vi "ATE_PwrMtr_Cal.vi"() -> ()   [LabVIEW 2009]
doc: "Use this template to build a producer/consumer design pattern with events to produce queue items. Use this design pattern instead of the User Interface Event Handler pattern for user interfaces when you want to execute code asynchronously in response to an event without slowing the user interface responsiveness."
uses:
  <vilib>/Analysis/NI_AALPro.lvlib
panel:
  in  "Sig Gen Test Point":T1(ring)
  out "Mean Diff":dbl format="%0.2f"
  out "Std Dev":dbl format="%0.2f"
  in  "Power Meter Test Point":T2(ring)
  in  "Calibrate-Atten":bool
  in  "Configuration 1":bool
  in  "Set SigGen":bool
  in  "70 dB":bool
  in  "121 dB":bool
  in  "Switches":bool
  in  "Calibrate-SG":bool
  in  "Stop":bool
  out "Output File":path
  out "SigGen - PwrMtr":cluster{dbl[], dbl[]}[](graph)
  out "ATE_Power_Cal":cluster{dbl[], dbl[]}[](graph)
  in  "Data Directory":string="/home/operator/ate/data/ate_cal"
  in  "ATE TABS":enum32{"Status", "Controls"}(tab)=enum."Controls"
  out "ATE Switch Status":T3
  out "121dB\nAttenuators":bool[](array[boolean])
  out "70dB\nAttenuators":bool[](array[boolean])
  out "Signal Generator Status":T4={"Frequency (GHz)"=0.0, "RF Power (dBm)"=0.0, "RF Power"=TRUE} {"RF Power (dBm)" format="%.2g"}
  out "Power (dBm)":dbl
  out "121 Verified":bool
  out "70 Verfied":bool
  out "Power Returned (dBm)":dbl format="%.3f"
  in  "ATE Switches":T5
  in  "121 dB Atten":i32=121 min=0 max=121 step=1
  in  "70 dB Attn":i32=70 min=0 max=70 step=10
  in  "Start dBm":dbl=-5.0
  in  "Steps":i32=21
  in  "Steps Size":dbl=1.0 min=0.1 max=2.0 step=0.1 format="%.1g"
  out "P-State":string
  out "C-State":string
  # "1 dB"
  # "2 dB"
  # "4 dB"
  # "4 dB"
  # "10 dB"
  # "20 dB"
  # "40 dB"
  # "40 dB"
  # "10 dB"
  # "20 dB"
  # "40 dB"
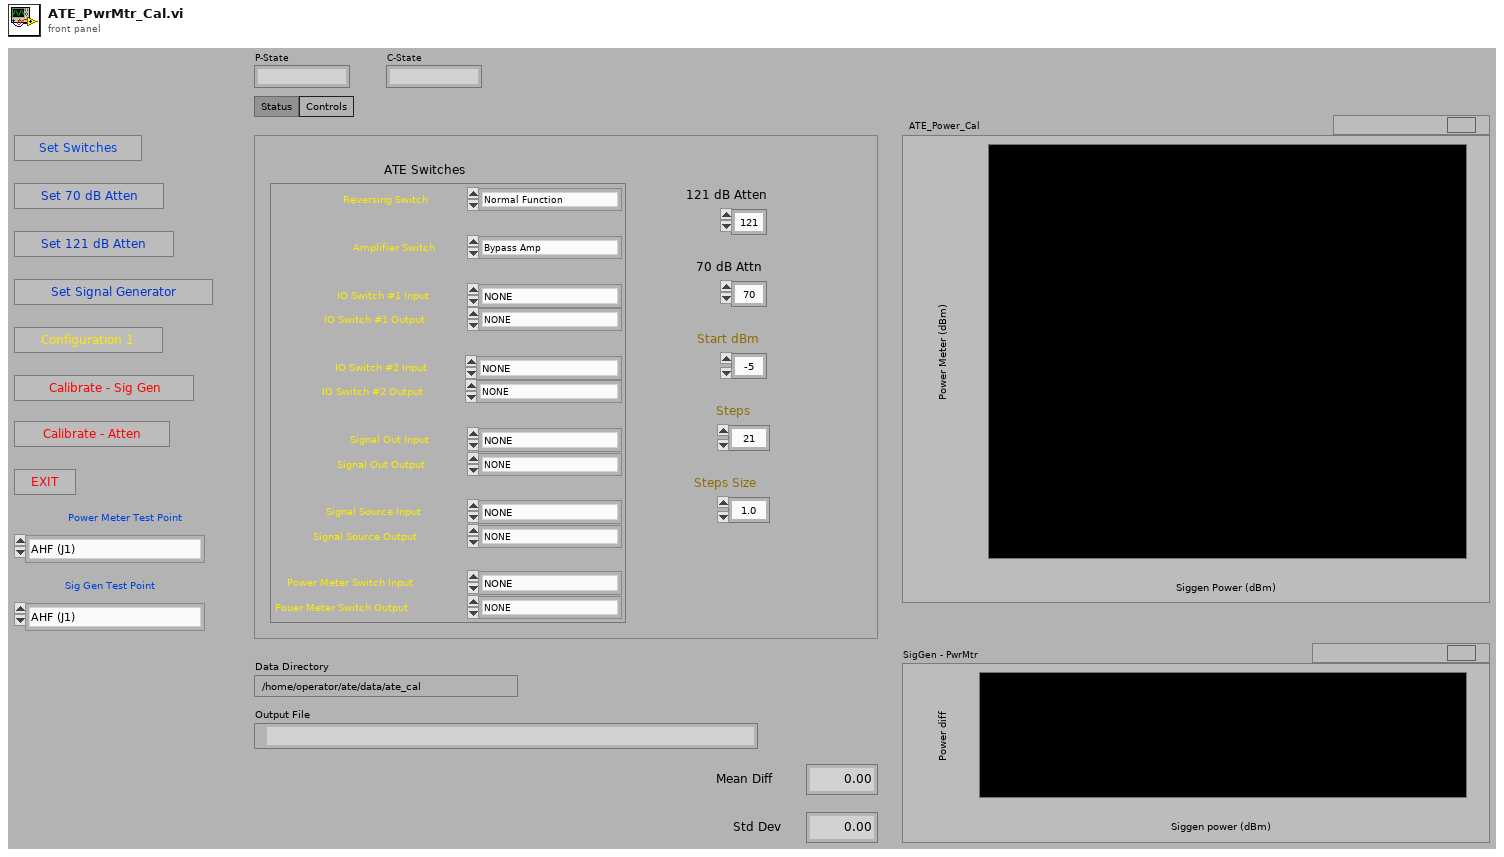
[diagram p1: front panel]
types:
  T1 = enum16{"AHF (J1)", "AHR (J2)", "AVR (J3)", "AVF (J4)", "NG1 (J5)", "Power Meter (J6)", "Sig Gen (J7)", "TXH-TXV Switch (J8)", "Power Meter Direct", ""}
  T2 = enum16{"AHF (J1)", "AHR (J2)", "AVR (J3)", "AVF (J4)", "NG1 (J5)", "Power Meter (J6)", "Sig Gen (J7)", "TXH-TXV Switch (J8)", "Sig Gen Direct"}
  T3 = cluster{"Reversing Switch ":bool, "IO Switch #1":bool, "IO Switch #2":bool, "Signal Out":bool, "Signal Source":bool, "Power Meter":bool, "Amp By Pass":bool}
  T4 = cluster{"Frequency (GHz)":dbl, "RF Power (dBm)":dbl, "RF Power":bool}
  T5 = cluster{"Reversing Switch":enum16{"Normal Function", "Reversing Function"}, "IO Switch #1 Input":enum16{"NONE", "AHR (J2)", "Splitter", "Signal Out Switch (S3)", "Reversing Switch"}, "IO Switch #1 Output":enum16{"NONE", "AHR (J2)", "Delay Device (S4)", "Power Meter Switch (S5)", "Reversing Switch"}, "IO Switch #2 Input":enum16{"NONE", "AVR (J3)", "Splitter", "Signal Out Switch (S3)", " 2W Term (TM1)", "Reversing Switch"}, "IO Switch #2 Output":enum16{"NONE", "AVR (J3)", "Signal Out Switch (S3)", "Power Meter Switch (S5)", "Reversing Switch", "2W Term (TM1)"}, "Signal Out Input":enum16{"NONE", "Amp Bypass Switch (S6)", "IO Switch #1 (S1)", "IO Switch #2 (S2)", "2W Term (TM3)"}, "Signal Out Output":enum16{"NONE", "2 Watt Term (TM3)", "Splitter", "Power Meter Switch (S5)"}, "Signal Source Input":enum16{"NONE", "Delay Device", "Signal Generator (J7)", "Inside Noise Box NF (J5)", "2W Term (TM3)"}, "Signal Source Output":enum16{"NONE", "Amp Bypass Switch", "Test Pulse Generator", "Power Meter Switch (S5)"}, "Power Meter Switch Input":enum16{"NONE", "IO Switch #1 (S1)", "Signal Source Switch (S4)", "Signal Out Switch (S3)", "IO Switch #2 (S2)", "TXH-TXV Switch (J8)"}, "Pouer Meter Switch Output":enum16{"NONE", "Power Meter (J6)"}, "Amplifier Switch":enum16{"Bypass Amp", "Include Amp"}}
  T6 = cluster{"Frequency (GHz)":dbl, "RF Power (dBm)":dbl, "RF ON/OFF":bool}
  T7 = enum16{"open", "replace", "create", "open or create", "replace or create", "replace or create with confirmation"}
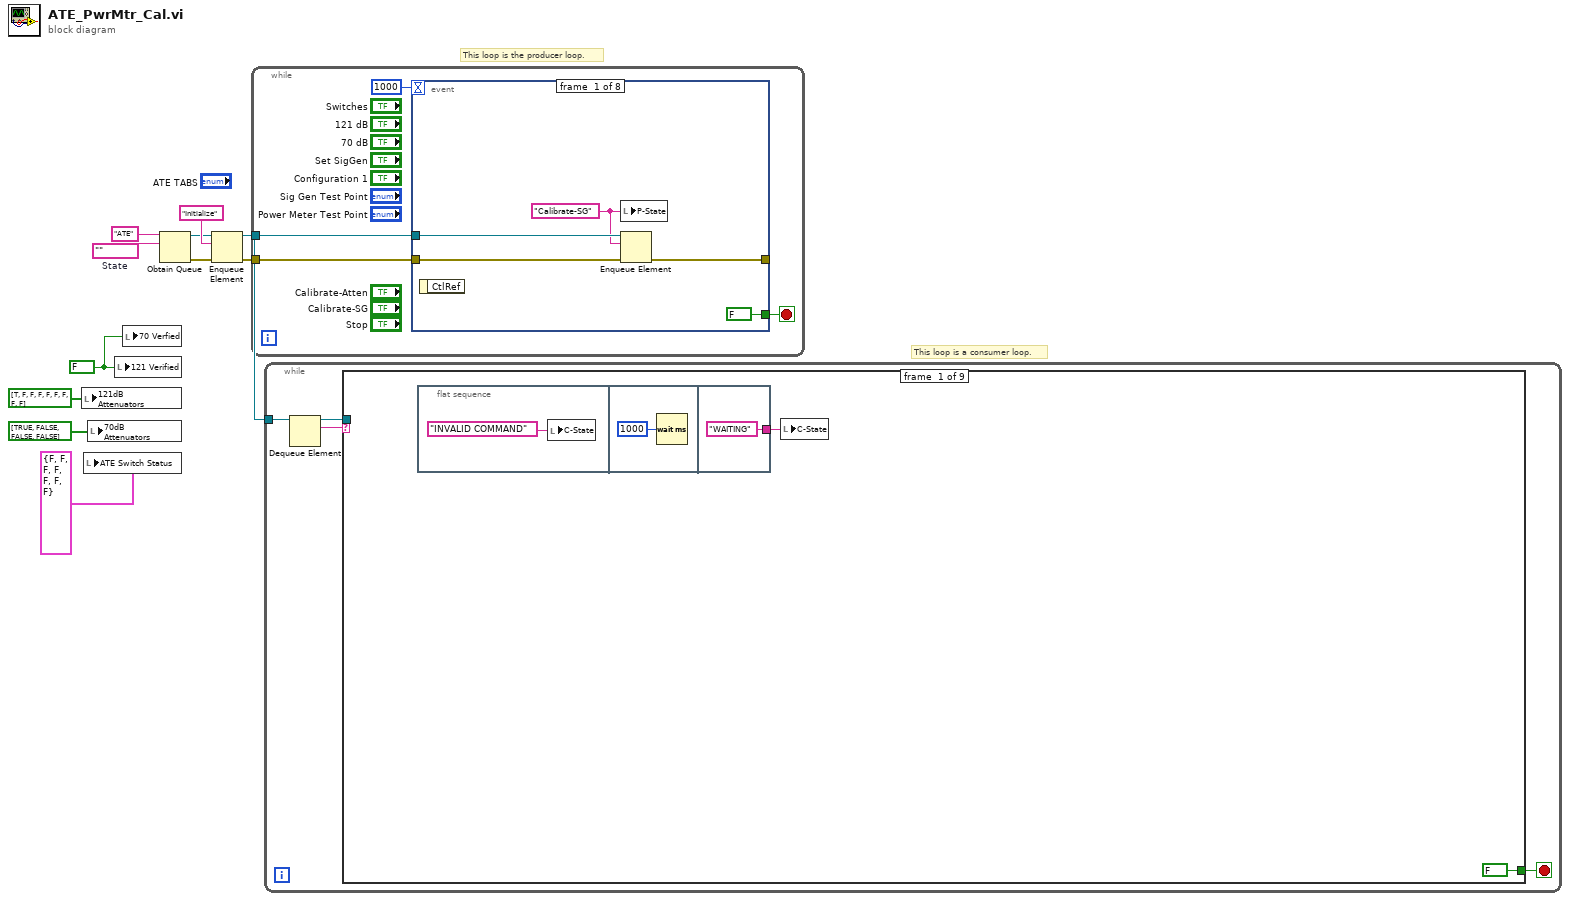
[diagram p0: block diagram]
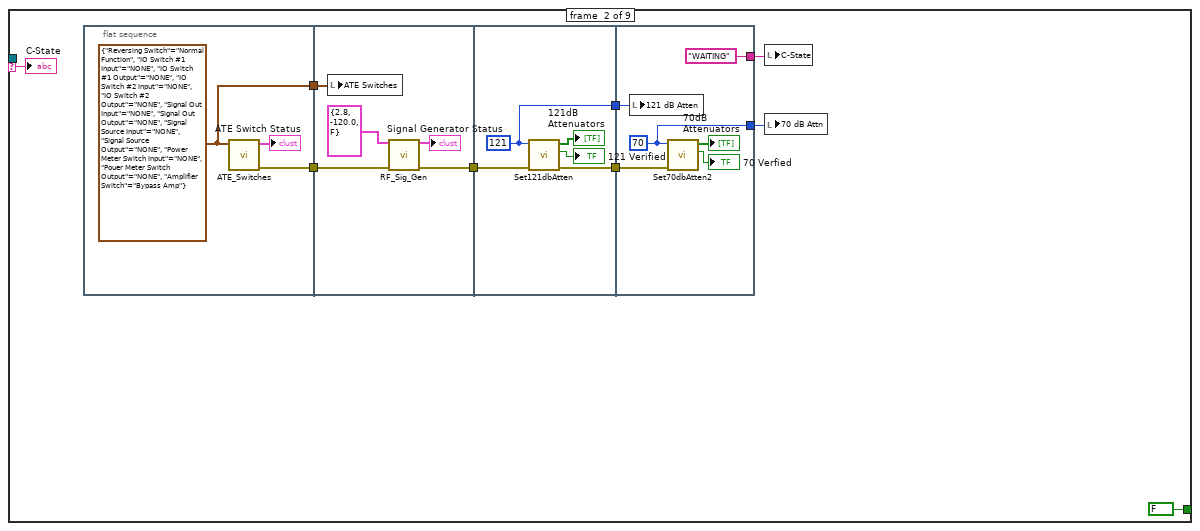
[diagram p2: hidden frame]
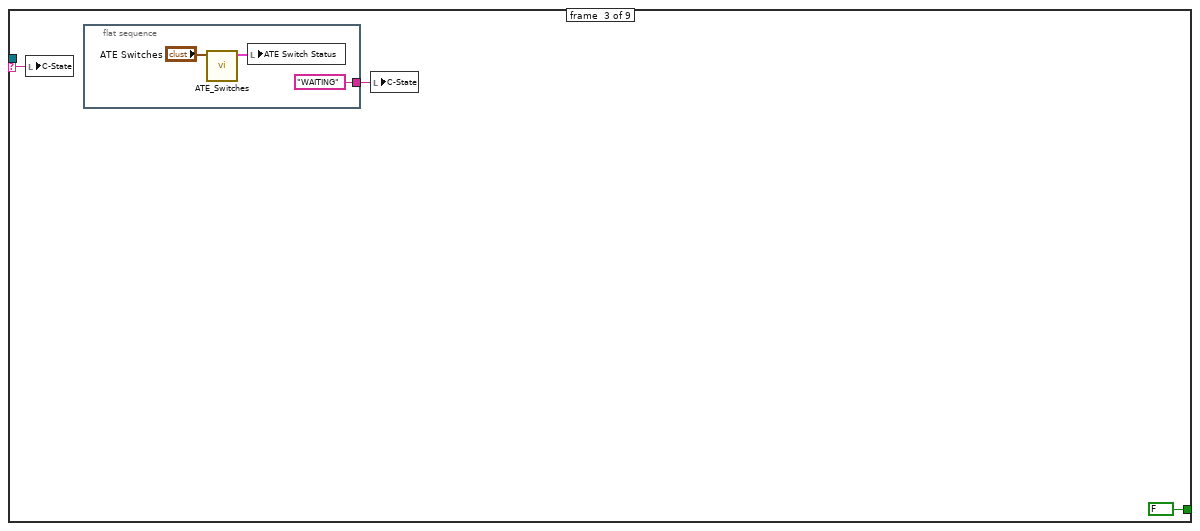
[diagram p3: hidden frame]
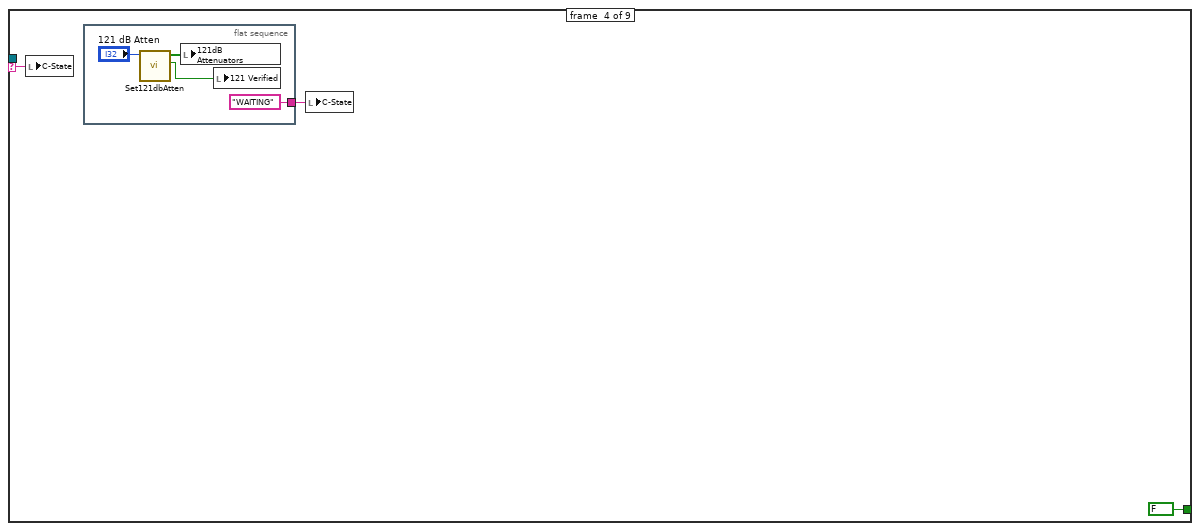
[diagram p4: hidden frame]
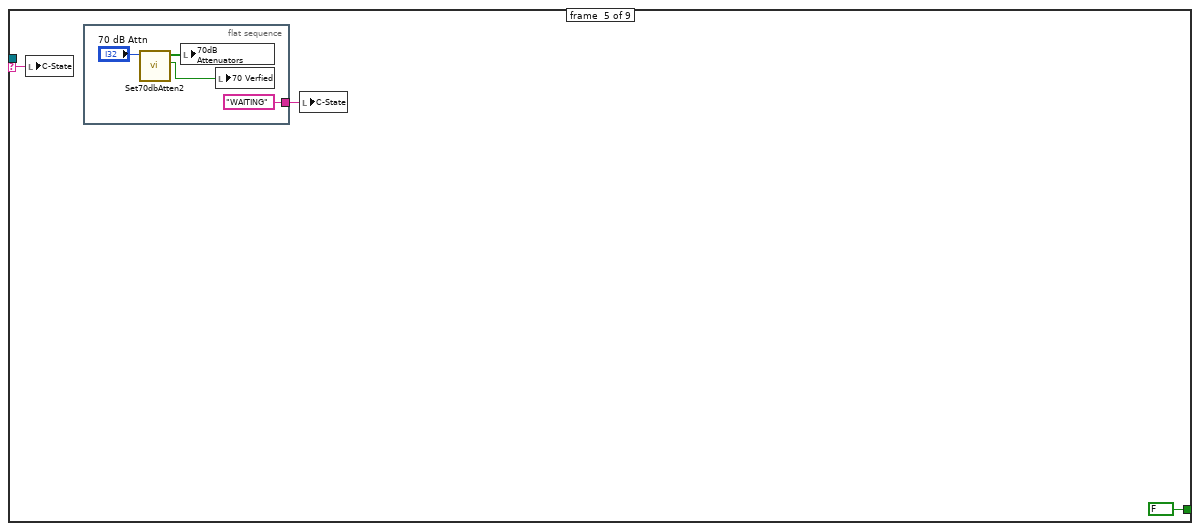
[diagram p5: hidden frame]
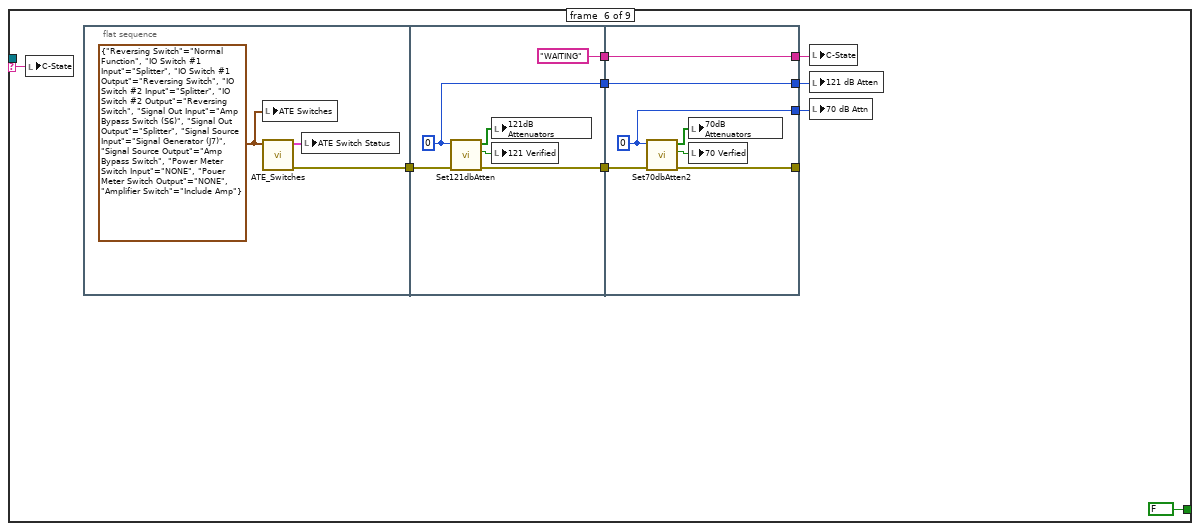
[diagram p6: hidden frame]
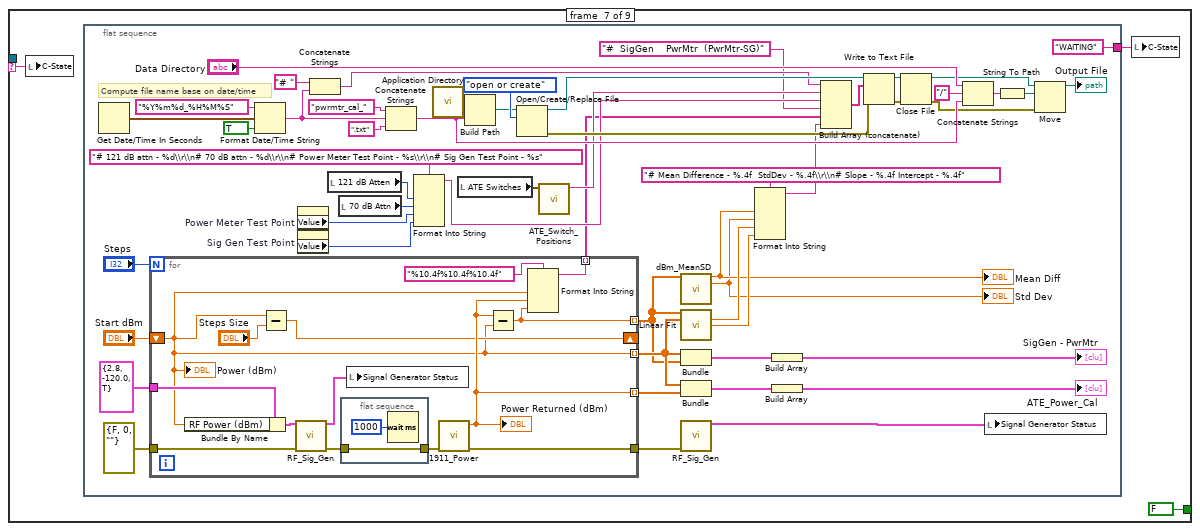
[diagram p7: hidden frame]
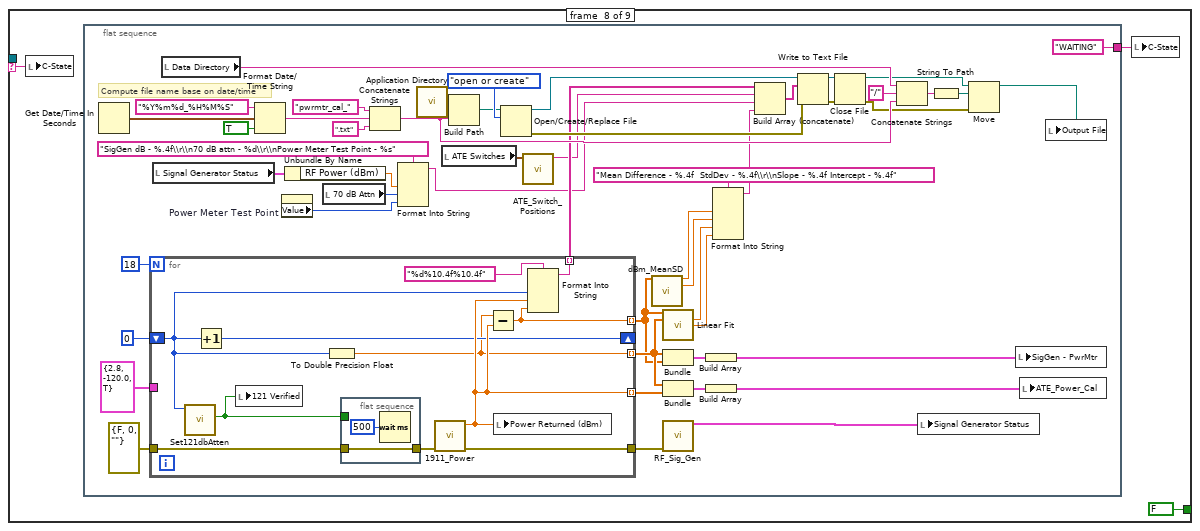
[diagram p8: hidden frame]
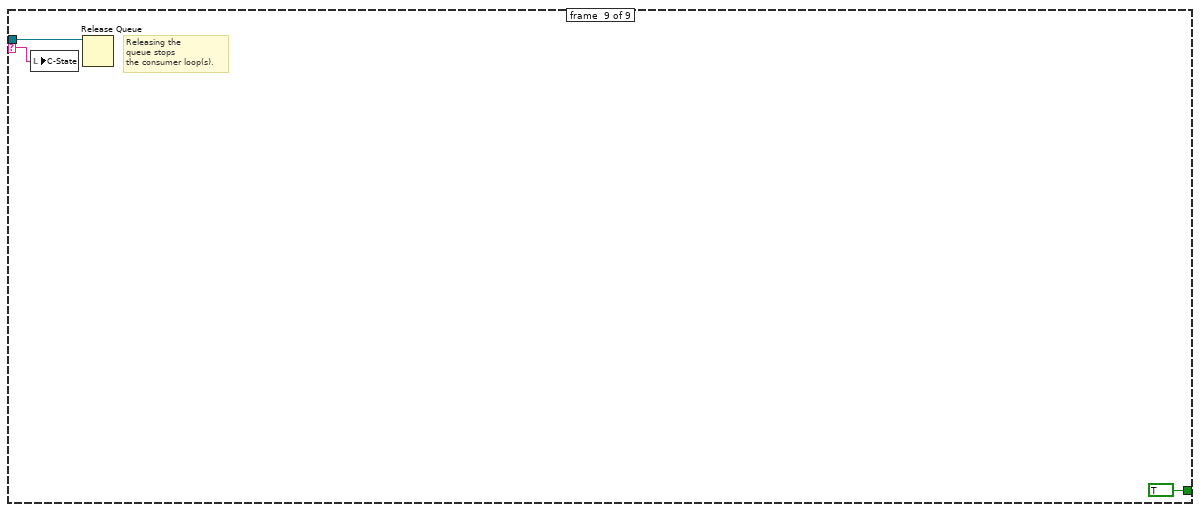
[diagram p9: hidden frame]
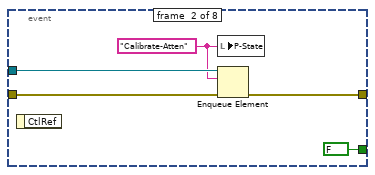
[diagram p10: hidden frame]
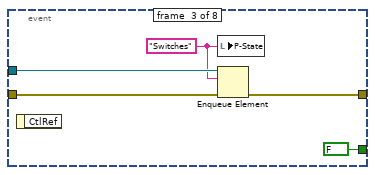
[diagram p11: hidden frame]
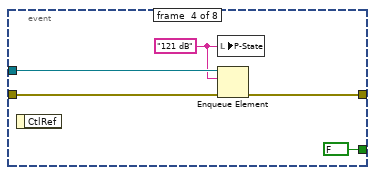
[diagram p12: hidden frame]
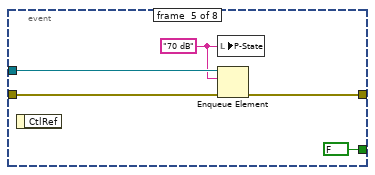
[diagram p13: hidden frame]
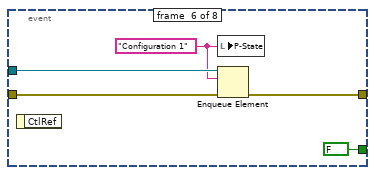
[diagram p14: hidden frame]
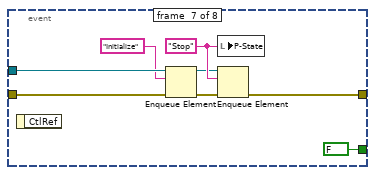
[diagram p15: hidden frame]
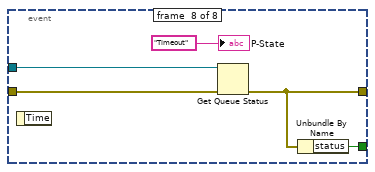
[diagram p16: hidden frame]
diagram:
  w1 = FALSE ("70 Verfied")
  w11 = ""  # State
  # "This loop is the producer loop."
  # "This loop is a consumer loop."
  n1 = local write "121dB\nAttenuators"(bool[] [TRUE, FALSE, FALSE, FALSE, FALSE, FALSE, FALSE, FALSE, FALSE] ("121dB\nAttenuators")) -> ()
  n2 = local write "ATE Switch Status"(T3 {"Reversing Switch "=FALSE, "IO Switch #1"=FALSE, "IO Switch #2"=FALSE, "Signal Out"=FALSE, "Signal Source"=FALSE, "Power Meter"=FALSE, "Amp By Pass"=FALSE} ("ATE Switch Status")) -> ()
  n3 = local write "70dB\nAttenuators"(bool[] [TRUE, FALSE, FALSE, FALSE] ("70dB\nAttenuators")) -> ()
  n4 = local write "121 Verified"(w1) -> ()
  n5 = local write "70 Verfied"(w1) -> ()
  n6 = Obtain Queue(name (unnamed)="ATE", element data type=w11) -> (queue out=w8:refnum<queue>, error out=w6:errorcluster)  [unwired: 3 in, 1 out]
  n7 = Enqueue Element(queue=w8, element="Initialize", error in (no error)=w6) -> (queue out=w7:refnum<queue>, error out=w5:errorcluster)  [unwired: 1 in, 1 out]
  n8 = while {
    tunnel: w7 -> [w15]
    tunnel: w5 -> [w14]
    stop <- w12 stop-if-true
    n9 = event shown="[6] \"Stop\": Value Change" {
      selector: _ -> [_ _ _ _ _ _ _ _]
      dyn-events: _ -> [_ _ _ _ _ _ _ _]
      timeout: 1000 -> [_ _ _ _ _ _ _ _]
      tunnel: w15 -> [w20 w25 w30 w35 w40 w45 w48 w58]
      tunnel: w14 -> [w19 w24 w29 w34 w39 w44 w50 w54]
      tunnel: [w18 w23 w28 w33 w38 w43 w53 w56] -> _
      tunnel: [FALSE FALSE FALSE FALSE FALSE FALSE FALSE w57] -> w12
      event #0 {
        w16 = "Calibrate-SG" ("element")
        n10 = event-data() -> ()  [unwired: 1 in, 1 out]
        n11 = local write "P-State"(w16) -> ()
        n12 = Enqueue Element(queue=w20, element=w16, error in (no error)=w19) -> (error out=w18:errorcluster)  [unwired: 1 in, 2 out]
      }
      event #1 {
        w21 = "Calibrate-Atten" ("element")
        n13 = event-data() -> ()  [unwired: 1 in, 1 out]
        n14 = local write "P-State"(w21) -> ()
        n15 = Enqueue Element(queue=w25, element=w21, error in (no error)=w24) -> (error out=w23:errorcluster)  [unwired: 1 in, 2 out]
      }
      event #2 {
        w26 = "Switches" ("element")
        n16 = event-data() -> ()  [unwired: 1 in, 1 out]
        n17 = local write "P-State"(w26) -> ()
        n18 = Enqueue Element(queue=w30, element=w26, error in (no error)=w29) -> (error out=w28:errorcluster)  [unwired: 1 in, 2 out]
      }
      event #3 {
        w31 = "121 dB" ("element")
        n19 = event-data() -> ()  [unwired: 1 in, 1 out]
        n20 = local write "P-State"(w31) -> ()
        n21 = Enqueue Element(queue=w35, element=w31, error in (no error)=w34) -> (error out=w33:errorcluster)  [unwired: 1 in, 2 out]
      }
      event #4 {
        w36 = "70 dB" ("element")
        n22 = event-data() -> ()  [unwired: 1 in, 1 out]
        n23 = local write "P-State"(w36) -> ()
        n24 = Enqueue Element(queue=w40, element=w36, error in (no error)=w39) -> (error out=w38:errorcluster)  [unwired: 1 in, 2 out]
      }
      event #5 {
        w41 = "Configuration 1" ("element")
        n25 = event-data() -> ()  [unwired: 1 in, 1 out]
        n26 = local write "P-State"(w41) -> ()
        n27 = Enqueue Element(queue=w45, element=w41, error in (no error)=w44) -> (error out=w43:errorcluster)  [unwired: 1 in, 2 out]
      }
      event #6 {
        w51 = "Stop" ("element")
        n28 = event-data() -> ()  [unwired: 1 in, 1 out]
        n29 = Enqueue Element(queue=w48, element="Initialize", error in (no error)=w50) -> (queue out=w47:refnum<queue>, error out=w49:errorcluster)  [unwired: 1 in, 1 out]
        n30 = local write "P-State"(w51) -> ()
        n31 = Enqueue Element(queue=w47, element=w51, error in (no error)=w49) -> (error out=w53:errorcluster)  [unwired: 1 in, 2 out]
      }
      event #7 {
        n32 = event-data() -> ()  [unwired: 1 in, 1 out]
        n33 = Get Queue Status(queue=w58, error in (no error)=w54) -> (error out=w56:errorcluster)  [unwired: 1 in, 7 out]
        n34 = Unbundle By Name(w56) -> ("status"=w57:bool)
        "P-State" <- "Timeout" ("element")
      }
    }
  }
  n35 = while {
    tunnel: w7 -> [w62]
    stop <- w59 stop-if-true
    n36 = Dequeue Element(queue=w62) -> (queue out=w60:refnum<queue>, element=w61:string)  [unwired: 2 in, 2 out]
    n37 = case shown="\"Calibrate-Atten\"" w61 {
      selector: w61 -> [_ w75 w98 w103 w110 w123 w142 w215 w282]
      tunnel: w60 -> [_ _ _ _ _ _ _ _ w281]
      tunnel: [FALSE FALSE FALSE FALSE FALSE FALSE FALSE FALSE TRUE] -> w59
      frame #0 {
        n38 = flat-sequence {
          tunnel: ["WAITING" ("element")] -> w63
          frame #0 {
            n39 = local write "C-State"("INVALID COMMAND" ("C-State")) -> ()
          }
          frame #1 {
            n40 = Wait (ms)(milliseconds to wait=u32 1000) -> ()  [unwired: 1 out]
          }
          frame #2 {
          }
        }
        n41 = local write "C-State"(w63) -> ()
      }
      frame #1 {
        n42 = flat-sequence {
          tunnel: [w78] -> w72
          tunnel: [w77] -> w70
          tunnel: w72 -> [w82]
          tunnel: [w81] -> w71
          tunnel: w70 -> [w80]
          tunnel: w71 -> [w88]
          tunnel: [w87] -> w73
          tunnel: [w86] -> w69
          tunnel: ["WAITING" ("element")] -> w74
          tunnel: w73 -> [w94]
          tunnel: w69 -> [w92]
          tunnel: [w90] -> w68
          frame #0 {
            w77 = T5 {"Reversing Switch"=enum."Normal Function", "IO Switch #1 Input"=enum."NONE", "IO Switch #1 Output"=enum."NONE", "IO Switch #2 Input"=enum."NONE", "IO Switch #2 Output"=enum."NONE", "Signal Out Input"=enum."NONE", "Signal Out Output"=enum."NONE", "Signal Source Input"=enum."NONE", "Signal Source Output"=enum."NONE", "Power Meter Switch Input"=enum."NONE", "Pouer Meter Switch Output"=enum."NONE", "Amplifier Switch"=enum."Bypass Amp"} ("ATE Switches")
            n43 = call "ATE_Switches.vi"("ATE Switches"=w77) -> ("Switch Errors"=w78:errorcluster, "ATE Switch Status"=→"ATE Switch Status":T3)  [unwired: 9 in]
          }
          frame #1 {
            n44 = local write "ATE Switches"(w80) -> ()
            n45 = call "RF_Sig_Gen.vi"("Signal Generator Control"=T6 {"Frequency (GHz)"=2.8, "RF Power (dBm)"=-120.0, "RF ON/OFF"=FALSE}, "error in"=w82) -> ("Signal Generator Status"=→"Signal Generator Status":T4, "Sig Gen Errors"=w81:errorcluster)  [unwired: 12 in]
          }
          frame #2 {
            w86 = 121 ("Attenuation (dB)")
            n46 = call "Set121dbAtten.vi"("error in (no error)"=w88, "Attenuation (dB)"=w86) -> ("error out"=w87:errorcluster, "Verfied"=→"121 Verified":bool, "Active Attenuators"=→"121dB\nAttenuators":bool[])  [unwired: 7 in]
          }
          frame #3 {
            w90 = 70 ("Attenuation (dB)")
            n47 = local write "121 dB Atten"(w92) -> ()
            n48 = call "Set70dbAtten2.vi"("error in (no error)"=w94, "Attenuation (dB)"=w90) -> ("Verfied"=→"70 Verfied":bool, "Active Attenuators"=→"70dB\nAttenuators":bool[])  [unwired: 7 in, 1 out]
          }
        }
        n49 = local write "C-State"(w74) -> ()
        n50 = local write "70 dB Attn"(w68) -> ()
        "C-State" <- w75
      }
      frame #2 {
        n51 = local write "C-State"(w98) -> ()
        n52 = flat-sequence {
          tunnel: ["WAITING" ("element")] -> w96
          frame #0 {
            n53 = call "ATE_Switches.vi"("ATE Switches"="ATE Switches") -> ("ATE Switch Status"=w100:T3)  [unwired: 9 in, 1 out]
            n54 = local write "ATE Switch Status"(w100) -> ()
          }
        }
        n55 = local write "C-State"(w96) -> ()
      }
      frame #3 {
        n56 = local write "C-State"(w103) -> ()
        n57 = flat-sequence {
          tunnel: ["WAITING" ("element")] -> w102
          frame #0 {
            n58 = call "Set121dbAtten.vi"("Attenuation (dB)"="121 dB Atten") -> ("Verfied"=w105:bool, "Active Attenuators"=w107:bool[])  [unwired: 8 in, 1 out]
            n59 = local write "121dB\nAttenuators"(w107) -> ()
            n60 = local write "121 Verified"(w105) -> ()
          }
        }
        n61 = local write "C-State"(w102) -> ()
      }
      frame #4 {
        n62 = local write "C-State"(w110) -> ()
        n63 = flat-sequence {
          tunnel: ["WAITING" ("element")] -> w109
          frame #0 {
            n64 = call "Set70dbAtten2.vi"("Attenuation (dB)"="70 dB Attn") -> ("Verfied"=w112:bool, "Active Attenuators"=w114:bool[])  [unwired: 8 in, 1 out]
            n65 = local write "70dB\nAttenuators"(w114) -> ()
            n66 = local write "70 Verfied"(w112) -> ()
          }
        }
        n67 = local write "C-State"(w109) -> ()
      }
      frame #5 {
        n68 = local write "C-State"(w123) -> ()
        n69 = flat-sequence {
          tunnel: [w127] -> w122
          tunnel: w122 -> [w133]
          tunnel: [w128] -> w120
          tunnel: ["WAITING" ("element")] -> w119
          tunnel: [w131] -> w118
          tunnel: [w137] -> _
          tunnel: [w139] -> w121
          tunnel: [w140] -> w117
          tunnel: w120 -> [w140]
          tunnel: w119 -> [w139]
          tunnel: w118 -> [w138]
          tunnel: [w136] -> w116
          frame #0 {
            w125 = T5 {"Reversing Switch"=enum."Normal Function", "IO Switch #1 Input"=enum."Splitter", "IO Switch #1 Output"=enum."Reversing Switch", "IO Switch #2 Input"=enum."Splitter", "IO Switch #2 Output"=enum."Reversing Switch", "Signal Out Input"=enum."Amp Bypass Switch (S6)", "Signal Out Output"=enum."Splitter", "Signal Source Input"=enum."Signal Generator (J7)", "Signal Source Output"=enum."Amp Bypass Switch", "Power Meter Switch Input"=enum."NONE", "Pouer Meter Switch Output"=enum."NONE", "Amplifier Switch"=enum."Include Amp"} ("ATE Switches")
            n70 = local write "ATE Switches"(w125) -> ()
            n71 = call "ATE_Switches.vi"("ATE Switches"=w125) -> ("Switch Errors"=w127:errorcluster, "ATE Switch Status"=w126:T3)  [unwired: 9 in]
            n72 = local write "ATE Switch Status"(w126) -> ()
          }
          frame #1 {
            w128 = 0 ("Attenuation (dB)")
            n73 = call "Set121dbAtten.vi"("error in (no error)"=w133, "Attenuation (dB)"=w128) -> ("error out"=w131:errorcluster, "Verfied"=w129:bool, "Active Attenuators"=w130:bool[])  [unwired: 7 in]
            n74 = local write "121dB\nAttenuators"(w130) -> ()
            n75 = local write "121 Verified"(w129) -> ()
          }
          frame #2 {
            w136 = 0 ("Attenuation (dB)")
            n76 = call "Set70dbAtten2.vi"("error in (no error)"=w138, "Attenuation (dB)"=w136) -> ("error out"=w137:errorcluster, "Verfied"=w135:bool, "Active Attenuators"=w134:bool[])  [unwired: 7 in]
            n77 = local write "70dB\nAttenuators"(w134) -> ()
            n78 = local write "70 Verfied"(w135) -> ()
          }
        }
        n79 = local write "C-State"(w121) -> ()
        n80 = local write "121 dB Atten"(w117) -> ()
        n81 = local write "70 dB Attn"(w116) -> ()
      }
      frame #6 {
        n82 = local write "C-State"(w142) -> ()
        n83 = flat-sequence {
          tunnel: ["WAITING" ("element")] -> w141
          frame #0 {
            # "Compute file name base on date/time"
            n84 = Get Date/Time In Seconds() -> (seconds since 1Jan1904=w192:timestamp)
            n85 = for {
              N: "Steps" -> [_]
              shift-right: [w199] -> _
              shift-left: "Start dBm" -> [w198]
              tunnel: errorcluster {"status"=FALSE, "code"=0, "source"=""} ("error out") -> [w208]
              tunnel: [w198] -> w163 mode=indexing
              tunnel: [w211] -> w149 mode=indexing
              tunnel: [w202] -> w162 mode=indexing
              tunnel: T6 {"Frequency (GHz)"=2.8, "RF Power (dBm)"=-120.0, "RF ON/OFF"=TRUE} ("Signal Generator Control") -> [w210]
              tunnel: [w204] -> w169
              tunnel: [w200] -> w168 mode=indexing
              n86 = Bundle By Name(cluster=w210, "RF Power (dBm)"=w198) -> (w209:T6)
              n87 = Subtract(x=w198, y="Steps Size") -> (x-y=w199:dbl)
              n88 = call "RF_Sig_Gen.vi"("Signal Generator Control"=w209, "error in"=w208) -> ("Signal Generator Status"=w206:T4, "Sig Gen Errors"=w207:errorcluster)  [unwired: 12 in]
              n89 = flat-sequence {
                tunnel: w207 -> [w212]
                tunnel: [w212] -> w205
                frame #0 {
                  n90 = Wait (ms)(milliseconds to wait=u32 1000) -> ()  [unwired: 1 out]
                }
              }
              n91 = local write "Signal Generator Status"(w206) -> ()
              n92 = call "1911_Power.vi"("error in (no error)"=w205) -> ("Error out"=w204:errorcluster, "Power returned (dBm)"=w200:dbl)  [unwired: 7 in]
              "Power Returned (dBm)" <- w200
              n93 = Subtract(x=w200, y=w198) -> (x-y=w202:dbl)
              n94 = Format Into String(format string="%10.4f%10.4f%10.4f", w198, w200, w202) -> (resulting string=w211:string)  [unwired: 2 in, 1 out]
              "Power (dBm)" <- w198
            }
            n95 = Format Date/Time String(time format string (%c)="%Y%m%d_%H%M%S", seconds (now)=w192, UTC format=TRUE) -> (date/time string=w153:string)
            n96 = property on="Power Meter Test Point" class="Enum (strict)"() -> ("Value"=w161:T2)  [unwired: 2 in, 2 out]
            n97 = property on="Sig Gen Test Point" class="Enum (strict)"() -> ("Value"=w145:T1)  [unwired: 2 in, 2 out]
            n98 = Concatenate Strings("# " ("string"), w153) -> (w152:string)
            n99 = local read "121 dB Atten"() -> (w165:i32)
            n100 = local read "70 dB Attn"() -> (w166:i32)
            n101 = Concatenate Strings("pwrmtr_cal_", w153, ".txt") -> (w174:string)
            n102 = Format Into String(format string="# 121 dB attn - %d\\r\\n# 70 dB attn - %d\\r\\n# Power Meter Test Point - %s\\r\\n# Sig Gen Test Point - %s", w165, w166, w161, w145) -> (resulting string=w150:string)  [unwired: 2 in, 1 out]
            n103 = call <vilib>:"Application Directory.vi"() -> ("Application Directory"=w191:path)
            n104 = local read "ATE Switches"() -> (w146:T5)
            n105 = Build Path(base path=w191, name or relative path=w174) -> (appended path=w182:path)
            n106 = Open/Create/Replace File(file path (use dialog)=w182, operation (0:open)=T7."open or create") -> (refnum out=w181:refnum<file>, error out=w180:errorcluster)  [unwired: 4 in, 1 out]
            n107 = call "ATE_Switch_Positions.vi"("ATE Switches"=w146) -> ("ATE Switch/Position"=w151:string)  [unwired: 10 in]
            n108 = call "dBm_MeanSD.vi"("dBm array"=w162) -> ("dBm mean"=w147:dbl, "Std Dev"=w144:dbl)  [unwired: 13 in]
            "Std Dev" <- w144
            "Mean Diff" <- w147
            n109 = call <vilib>:"Linear Fit.vi"("Y"=w162, "X"=w163) -> ("slope"=w156:dbl, "intercept"=w155:dbl)  [unwired: 9 in, 3 out]
            n110 = Bundle(w163, w162) -> (w186:cluster{dbl[], dbl[]})  [unwired: 1 in]
            n111 = Bundle(w163, w168) -> (w185:cluster{dbl[], dbl[]})  [unwired: 1 in]
            n112 = call "RF_Sig_Gen.vi"("error in"=w169) -> ("Signal Generator Status"=w170:T4)  [unwired: 13 in, 1 out]
            n113 = Format Into String(format string="# Mean Difference - %.4f  StdDev - %.4f\\r\\n# Slope - %.4f Intercept - %.4f", w147, w144, w156, w155) -> (resulting string=w159:string)  [unwired: 2 in, 1 out]
            n114 = Build Array(w186) -> (→"SigGen - PwrMtr":cluster{dbl[], dbl[]}[])
            n115 = Build Array(w185) -> (→"ATE_Power_Cal":cluster{dbl[], dbl[]}[])
            n116 = Build Array (concatenate)(w152, w151, w150, "#  SigGen    PwrMtr  (PwrMtr-SG)" ("format string"), w149, w159) -> (w160:string[])
            n117 = Write to Text File(file (use dialog)=w181, text=w160, error in=w180) -> (refnum out=w179:refnum<file>, error out=w178:errorcluster)  [unwired: 1 in, 1 out]
            n118 = Close File(refnum=w179, error in=w178) -> (path=w173:path, error out=w157:errorcluster)
            n119 = Concatenate Strings("Data Directory", "/" ("string"), w174) -> (w176:string)
            n120 = local write "Signal Generator Status"(w170) -> ()
            n121 = String To Path(string=w176) -> (path=w172:path)
            n122 = Move(source path=w173, error in=w157, 10:w172) -> (3:→"Output File":path)  [unwired: 2 in, 2 out]
          }
        }
        n123 = local write "C-State"(w141) -> ()
      }
      frame #7 {
        n124 = local write "C-State"(w215) -> ()
        n125 = flat-sequence {
          tunnel: ["WAITING" ("element")] -> w214
          frame #0 {
            # "Compute file name base on date/time"
            n126 = Get Date/Time In Seconds() -> (seconds since 1Jan1904=w236:timestamp)
            n127 = for {
              N: 18 -> [_]
              shift-right: [w271] -> _
              shift-left: 0 -> [w269]
              tunnel: errorcluster {"status"=FALSE, "code"=0, "source"=""} ("error out") -> [w272]
              tunnel: [w270] -> w251 mode=indexing
              tunnel: [w278] -> w254 mode=indexing
              tunnel: [w274] -> w250 mode=indexing
              tunnel: T6 {"Frequency (GHz)"=2.8, "RF Power (dBm)"=-120.0, "RF ON/OFF"=TRUE} ("Signal Generator Control") -> [_]
              tunnel: [w276] -> w256
              tunnel: [w273] -> w255 mode=indexing
              n128 = call "Set121dbAtten.vi"("Attenuation (dB)"=w269) -> ("Verfied"=w268:bool)  [unwired: 8 in, 2 out]
              n129 = Increment(x=w269) -> (x+1=w271:i32)
              n130 = local write "121 Verified"(w268) -> ()
              n131 = To Double Precision Float(number=w269) -> (double precision float=w270:dbl)
              n132 = flat-sequence {
                tunnel: [w279] -> w277
                tunnel: w272 -> [w279]
                tunnel: w268 -> [_]
                frame #0 {
                  n133 = Wait (ms)(milliseconds to wait=u32 500) -> ()  [unwired: 1 out]
                }
              }
              n134 = call "1911_Power.vi"("error in (no error)"=w277) -> ("Error out"=w276:errorcluster, "Power returned (dBm)"=w273:dbl)  [unwired: 7 in]
              n135 = Subtract(x=w270, y=w273) -> (x-y=w274:dbl)
              n136 = local write "Power Returned (dBm)"(w273) -> ()
              n137 = Format Into String(format string="%d%10.4f%10.4f", w269, w273, w274) -> (resulting string=w278:string)  [unwired: 2 in, 1 out]
            }
            n138 = local read "Signal Generator Status"() -> (w228:T4)
            n139 = local read "Data Directory"() -> (w244:string)
            n140 = Format Date/Time String(time format string (%c)="%Y%m%d_%H%M%S", seconds (now)=w236, UTC format=TRUE) -> (date/time string=w239:string)
            n141 = property on="Power Meter Test Point" class="Enum (strict)"() -> ("Value"=w229:T2)  [unwired: 2 in, 2 out]
            n142 = Unbundle By Name(w228) -> ("RF Power (dBm)"=w227:dbl)
            n143 = local read "70 dB Attn"() -> (w231:i32)
            n144 = Concatenate Strings("pwrmtr_cal_", w239, ".txt") -> (w258:string)
            n145 = Format Into String(format string="SigGen dB - %.4f\\r\\n70 dB attn - %d\\r\\nPower Meter Test Point - %s", w227, w231, w229) -> (resulting string=w252:string)  [unwired: 2 in, 1 out]
            n146 = call <vilib>:"Application Directory.vi"() -> ("Application Directory"=w235:path)
            n147 = local read "ATE Switches"() -> (w232:T5)
            n148 = Build Path(base path=w235, name or relative path=w258) -> (appended path=w233:path)
            n149 = Open/Create/Replace File(file path (use dialog)=w233, operation (0:open)=T7."open or create") -> (refnum out=w260:refnum<file>, error out=w259:errorcluster)  [unwired: 4 in, 1 out]
            n150 = call "ATE_Switch_Positions.vi"("ATE Switches"=w232) -> ("ATE Switch/Position"=w253:string)  [unwired: 10 in]
            n151 = call "dBm_MeanSD.vi"("dBm array"=w250) -> ("dBm mean"=w249:dbl, "Std Dev"=w217:dbl)  [unwired: 13 in]
            n152 = call <vilib>:"Linear Fit.vi"("Y"=w250, "X"=w251) -> ("slope"=w246:dbl, "intercept"=w245:dbl)  [unwired: 9 in, 3 out]
            n153 = Bundle(w251, w250) -> (w262:cluster{dbl[], dbl[]})  [unwired: 1 in]
            n154 = Bundle(w251, w255) -> (w261:cluster{dbl[], dbl[]})  [unwired: 1 in]
            n155 = call "RF_Sig_Gen.vi"("error in"=w256) -> ("Signal Generator Status"=w257:T4)  [unwired: 13 in, 1 out]
            n156 = Build Array(w262) -> (w242:cluster{dbl[], dbl[]}[])
            n157 = Build Array(w261) -> (w243:cluster{dbl[], dbl[]}[])
            n158 = Format Into String(format string="Mean Difference - %.4f  StdDev - %.4f\\r\\nSlope - %.4f Intercept - %.4f", w249, w217, w246, w245) -> (resulting string=w248:string)  [unwired: 2 in, 1 out]
            n159 = Build Array (concatenate)(w254, w253, w252, w248) -> (w220:string[])
            n160 = Write to Text File(file (use dialog)=w260, text=w220, error in=w259) -> (refnum out=w226:refnum<file>, error out=w225:errorcluster)  [unwired: 1 in, 1 out]
            n161 = Close File(refnum=w226, error in=w225) -> (path=w222:path, error out=w219:errorcluster)
            n162 = Concatenate Strings(w244, "/" ("string"), w258) -> (w223:string)
            n163 = local write "Signal Generator Status"(w257) -> ()
            n164 = String To Path(string=w223) -> (path=w221:path)
            n165 = Move(source path=w222, error in=w219, 10:w221) -> (3:w218:path)  [unwired: 2 in, 2 out]
            n166 = local write "SigGen - PwrMtr"(w242) -> ()
            n167 = local write "ATE_Power_Cal"(w243) -> ()
            n168 = local write "Output File"(w218) -> ()
          }
        }
        n169 = local write "C-State"(w214) -> ()
      }
      frame #8 {
        # "Releasing the\nqueue stops\nthe consumer loop(s)."
        n170 = local write "C-State"(w282) -> ()
        n171 = Release Queue(queue=w281) -> ()  [unwired: 2 in, 3 out]
      }
    }
  }
